vi "OCR_MakeTrainingbox.vi"(8 "error in (no error)":errorcluster, 11 "Image Name":string="tesseract") -> (0 "error out":errorcluster, 1 "standard error":string, 2 "standard output":string, 3 "error":bool)   [LabVIEW 2019]
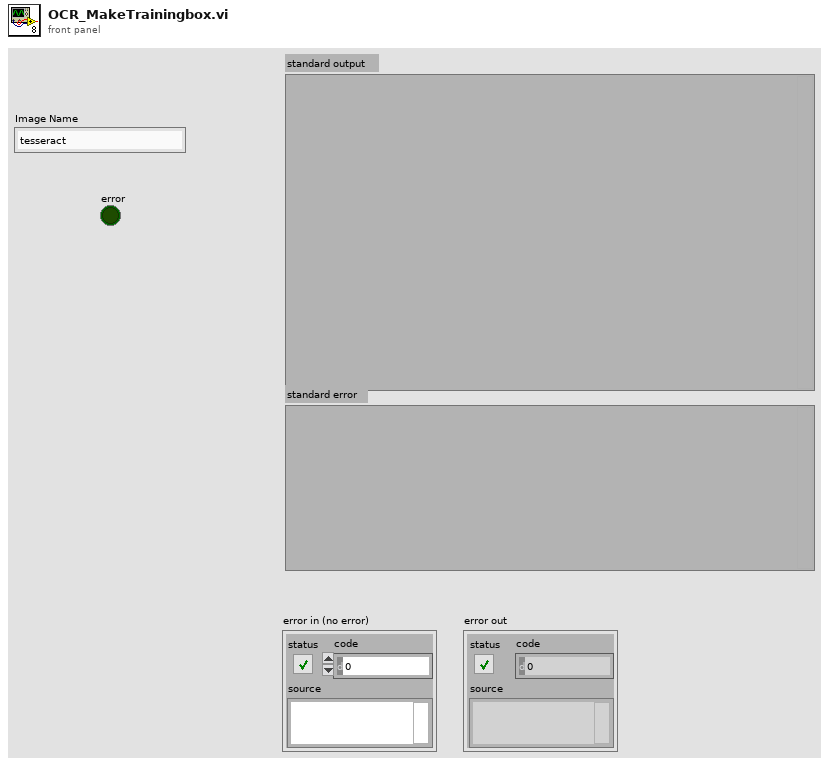
[diagram p1: front panel]
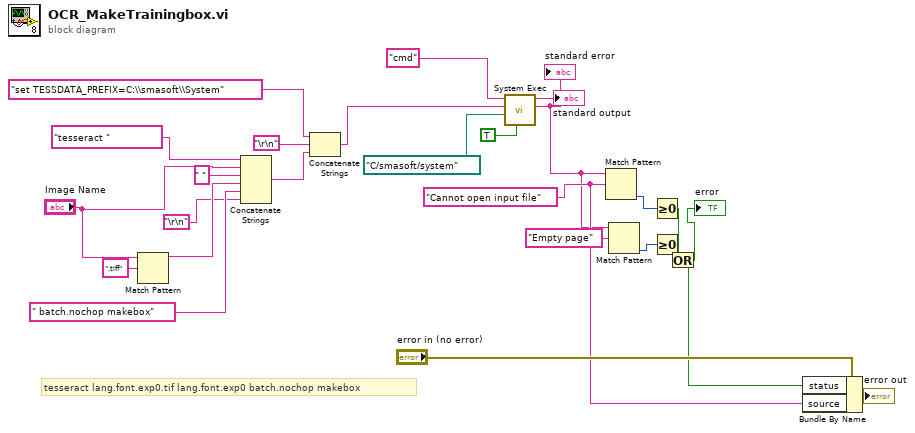
[diagram p0: block diagram]
diagram:
  w7 = "Cannot open input file" ("regular expression")
  # "tesseract lang.font.exp0.tif lang.font.exp0 batch.nochop makebox"
  n1 = Match Pattern(string="Image Name", regular expression=".tiff") -> (before substring=w15:string)  [unwired: 1 in, 3 out]
  n2 = Concatenate Strings("tesseract " ("standard input"), "Image Name", " " ("string"), w15, " batch.nochop makebox" ("regular expression"), "\r\n") -> (w12:string)
  n3 = Concatenate Strings("set TESSDATA_PREFIX=C:\\smasoft\\System" ("standard input"), "\r\n", w12) -> (w11:string)
  n4 = call <vilib>:"System Exec.vi"("run minimized? (F)"=TRUE, "working directory"=path "C:/smasoft/system", "standard input"=w11, "command line"="cmd") -> ("standard error"=w5:string, "standard output"=→"standard output":string)  [unwired: 4 in, 2 out]
  "standard error" <- w5
  n5 = Match Pattern(string=w5, regular expression=w7) -> (offset past match=w10:i32)  [unwired: 1 in, 3 out]
  n6 = Match Pattern(string=w5, regular expression="Empty page") -> (offset past match=w3:i32)  [unwired: 1 in, 3 out]
  n7 = Greater Or Equal To 0?(x=w10) -> (x >= 0?=w8:bool)
  n8 = Greater Or Equal To 0?(x=w3) -> (x >= 0?=w2:bool)
  n9 = Or(x=w8, y=w2) -> (x .or. y?=w1:bool)
  "error" <- w1
  n10 = Bundle By Name(cluster="error in (no error)", "status"=w1, "source"=w7) -> (→"error out":errorcluster)
